vi "Config Control Limits.vi"(0 "VISA resource name":refnum<visa-resource-name>, 1 "Threshold (0.0000)":dbl min=0.0 max=100.0 step=0.0001 format="%.4f", 2 "Reading must\nStay in Band (0s)":dbl min=0.0 max=86400.0 step=1.0, 5 "Loop (0: 1)":u16(ring) items=["1", "2"], 7 "Setpoint Limit (475.000)":dbl=475.0 min=0.0 max=1500.0 step=0.001 format="%.3f", 9 "Max Heater\nCurrent (0: 0.25A)":u16(ring) items=["0.25A", "0.5A", "1.0A", "2.0A"], 11 "error in (no error)":errorcluster, 12 "Positive Slope (0.0)":dbl min=0.0 max=100.0 step=0.1 format="%.1f", 13 "Negative Slope (0.0)":dbl min=0.0 max=100.0 step=0.1 format="%.1f", 14 "Max Heater\nRange (0: Off)":u16(ring) items=["Off", "1", "2", "3", "4", "5"]) -> (4 "VISA resource name out":refnum<visa-resource-name>, 15 "error out":errorcluster)   [LabVIEW 2025, in "Lake Shore Cryotronics 340.lvlib"]
doc: "This VI Configures the parameters of a control loop's limits and loop 1's settle parameters."
uses:
  Lake Shore Cryotronics 340.lvlib
panel:
  # "Control Loop Parameters"
  # "Loop 1 Settle Parameters"
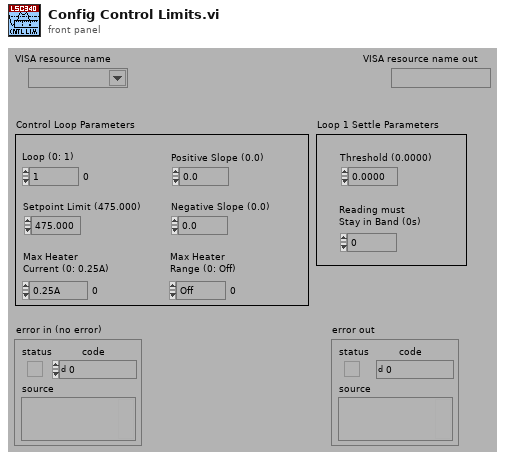
[diagram p1: front panel]
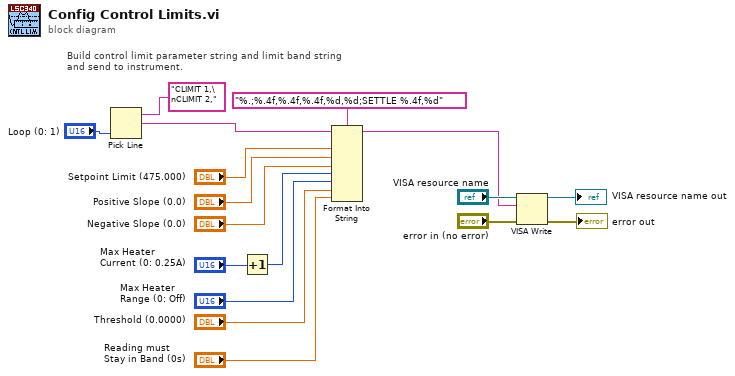
[diagram p0: block diagram]
diagram:
  # "Build control limit parameter string and limit band string\nand send to instrument."
  n1 = Pick Line(multi-line string="CLIMIT 1,\nCLIMIT 2,", line index="Loop (0: 1)") -> (output string=w10:string)  [unwired: 1 in]
  n2 = Increment(x="Max Heater\nCurrent (0: 0.25A)") -> (x+1=w6:u16)
  n3 = Format Into String(format string="%.;%.4f,%.4f,%.4f,%d,%d;SETTLE %.4f,%d", initial string=w10, "Setpoint Limit (475.000)", "Positive Slope (0.0)", "Negative Slope (0.0)", w6, "Max Heater\nRange (0: Off)", "Threshold (0.0000)", "Reading must\nStay in Band (0s)") -> (resulting string=w1:string)  [unwired: 1 in, 1 out]
  n4 = VISA Write(VISA resource name="VISA resource name", write buffer=w1, error in (no error)="error in (no error)") -> (VISA resource name out=→"VISA resource name out":refnum<visa-resource-name>, error out=→"error out":errorcluster)  [unwired: 1 out]
